vi "tarcfg serialize test.vi"() -> ()   [LabVIEW 2013, in "configuration tests.lvlib"]
uses:
  configuration tests.lvlib
  <vilib>/NI/Tag Bus Module Framework/root configuration/TBM configuration.lvclass
  Framework Configuration Classes/target configuration/PL_Target Configuration.lvclass
  <vilib>/NI/Tag Bus Module Framework/root configuration/Target Types.ctl
panel:
  out "pathok":bool
  out "OSok":bool
  out "nameok":bool
  out "hostok":bool
  out "classok":bool
  out "idok":bool
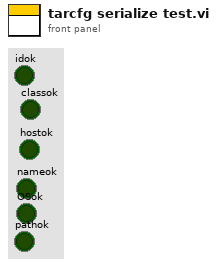
[diagram p1: front panel]
types:
  T1 = typedef "TBM configuration.lvclass/Target Types.ctl" = enum16{"Windows", "Mac", "Linux", "Linux RT ARM", "VxWorks", "Pharlap", "Other", "Linux RT x64"}
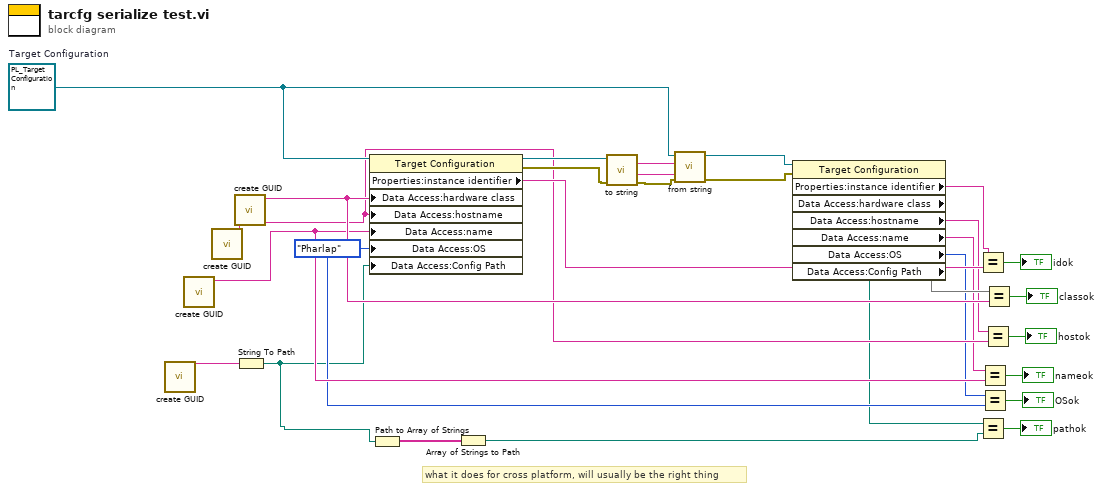
[diagram p0: block diagram]
diagram:
  w5 = Target_Types."Pharlap" ("OS")
  w14 = refnum<class "PL_Target Configuration.lvclass"> refnum  # Target Configuration
  # "what it does for cross platform, will usually be the right thing"
  n1 = call <vilib>:"create GUID.vi"() -> ("uuid"=w13:string)  [unwired: 11 in]
  n2 = call <vilib>:"create GUID.vi"() -> ("uuid"=w17:string)  [unwired: 11 in]
  n3 = call <vilib>:"create GUID.vi"() -> ("uuid"=w10:string)  [unwired: 11 in]
  n4 = call <vilib>:"create GUID.vi"() -> ("uuid"=w18:string)  [unwired: 11 in]
  n5 = String To Path(string=w13) -> (path=w3:path)
  n6 = property class="Target Configuration"(reference=w14, "Data Access:hardware class"=w18, "Data Access:hostname"=w10, "Data Access:name"=w17, "Data Access:OS"=w5, "Data Access:Config Path"=w3) -> (reference out=w27:refnum<class "PL_Target Configuration.lvclass">, error out=w16:errorcluster, "Properties:instance identifier"=w23:string)  [unwired: 1 in]
  n7 = Path to Array of Strings(0:w3) -> (2:w2:string[])  [unwired: 1 out]
  n8 = Array of Strings to Path(0:w2) -> (2:w1:path)  [unwired: 1 in]
  n9 = call-dynamic "to string.vi"("error in"=w16, "configuration in"=w27) -> ("error out"=w15:errorcluster, "data"=w28:string, "version"=w29:string)  [unwired: 6 in, 1 out]
  n10 = call-dynamic "from string.vi"("error in"=w15, "data"=w28, "version"=w29, "configuration in"=w14) -> ("error out"=w26:errorcluster, "configuration out"=w25:refnum<class "PL_Target Configuration.lvclass">)  [unwired: 6 in]
  n11 = property class="Target Configuration"(reference=w25, error in=w26) -> ("Properties:instance identifier"=w24:string, "Data Access:hardware class"=w12, "Data Access:hostname"=w11:string, "Data Access:name"=w9:string, "Data Access:OS"=w6:T1, "Data Access:Config Path"=w4:path)  [unwired: 2 out]
  n12 = Equal?(x=w24, y=w23) -> (x = y?=→"idok":bool)
  n13 = Equal?(x=w4, y=w1) -> (x = y?=→"pathok":bool)
  n14 = Equal?(x=w9, y=w17) -> (x = y?=→"nameok":bool)
  n15 = Equal?(x=w6, y=w5) -> (x = y?=→"OSok":bool)
  n16 = Equal?(x=w11, y=w10) -> (x = y?=→"hostok":bool)
  n17 = Equal?(x=w12, y=w18) -> (x = y?=→"classok":bool)
